vi "Program11.vi"() -> ()   [LabVIEW 2020]
panel:
  out "Y":dbl
  in  "X":dbl
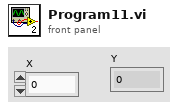
[diagram p1: front panel]
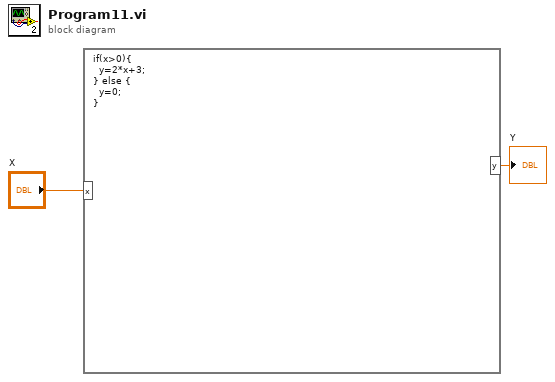
[diagram p0: block diagram]
diagram:
  n1 = formula code="if(x>0){\n  y=2*x+3;\n} else {\n  y=0;\n}"("x"="X") -> ("y"=→"Y":dbl)
